vi "Convert Configuration Variant.vi"(11 "Current Configuration":variant) -> (1 "Used Defaults":bool, 2 "Converted Old Version":bool, 3 "Configuration":T1)   [LabVIEW 2020, in "Logger.lvlib" / "Configuration.lvclass"]
doc: "This VI handles conversion of configuration data from variant, including handling possible changes to the configuration format.\n____\nPeloton Config 2.0.0.9\nCopyright (c) 2024, Peloton"
uses:
  Configuration.lvclass
  Configuration--cluster.ctl
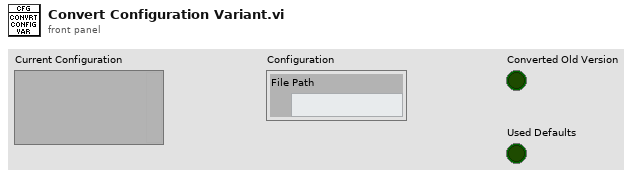
[diagram p1: front panel]
types:
  T1 = typedef "Logger.lvlib/Configuration.lvclass/Configuration--cluster.ctl" = cluster{"File Path":path}
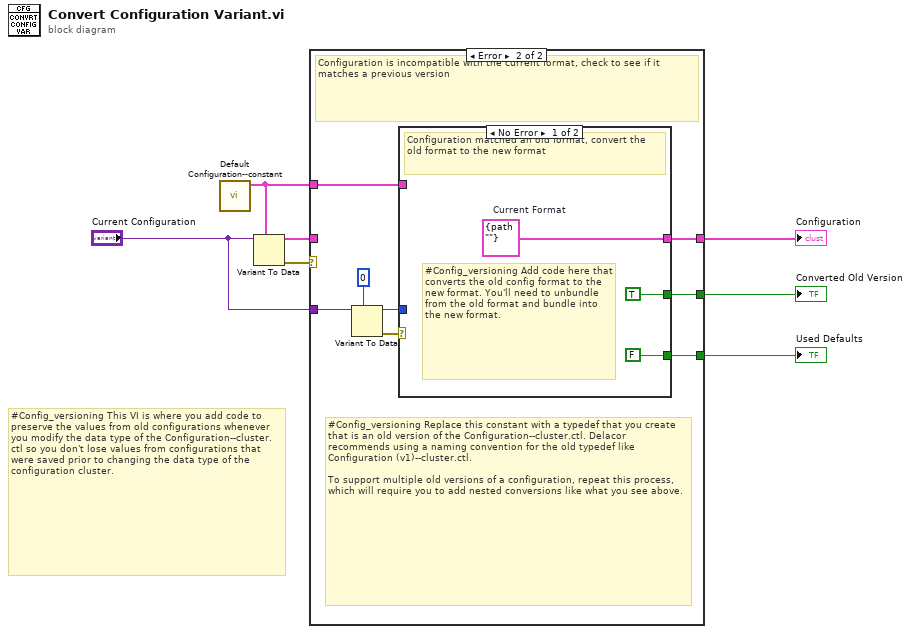
[diagram p0: block diagram]
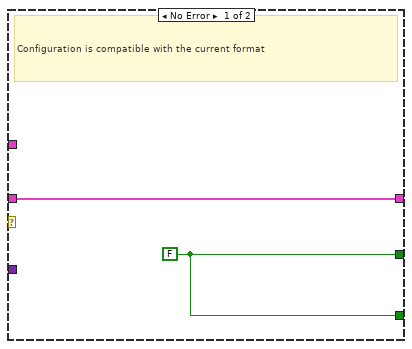
[diagram p2: hidden frame]
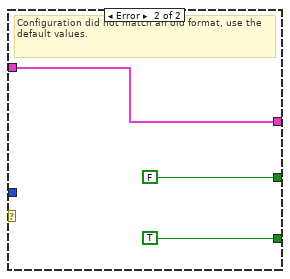
[diagram p3: hidden frame]
diagram:
  # "#Config_versioning This VI is where you add code to preserve the values from old configurations whenever you modify the data type of the Configuration--cluster.ctl so you don't lose values from configurations that were saved prior to changing the data type of the configuration cluster."
  n1 = call "Default Configuration--constant.vi"() -> ("Default Configuration"=w1:T1)  [unwired: 11 in]
  n2 = Variant To Data(type=w1, Variant="Current Configuration") -> (data=w6:T1, error out=w7:errorcluster)  [unwired: 1 in]
  n3 = case shown="Error" w7 {
    tunnel: w6 -> [w9 _]
    tunnel: [w9 w13] -> w5
    tunnel: [w8 w12] -> w4
    tunnel: [w8 w11] -> w3
    tunnel: "Current Configuration" -> [_ w17]
    tunnel: w1 -> [_ w14]
    frame No Error {
      w8 = FALSE
      # "Configuration is compatible with the current format"
    }
    frame Error {
      # "#Config_versioning Replace this constant with a typedef that you create that is an old version of the Configuration--cluster.ctl. Delacor recommends using a naming convention for the old typedef like Configuration (v1)--cluster.ctl.\n\nTo support multiple old versions of a configuration, repeat this process, which will require you to add nested conversions like what you see above."
      # "Configuration is incompatible with the current format, check to see if it matches a previous version"
      n4 = Variant To Data(type=0, Variant=w17) -> (data=w15:i32, error out=w16:errorcluster)  [unwired: 1 in]
      n5 = case shown="No Error" w16 {
        tunnel: w15 -> [_ _]
        tunnel: w14 -> [_ w23]
        tunnel: [w20 w23] -> w13
        tunnel: [TRUE FALSE] -> w12
        tunnel: [FALSE TRUE] -> w11
        frame No Error {
          w20 = T1 {"File Path"=path ""}  # Current Format
          # "#Config_versioning Add code here that converts the old config format to the new format. You'll need to unbundle from the old format and bundle into the new format."
          # "Configuration matched an old format, convert the old format to the new format"
        }
        frame Error {
          # "Configuration did not match an old format, use the default values."
        }
      }
    }
  }
  "Configuration" <- w5
  "Converted Old Version" <- w4
  "Used Defaults" <- w3
